vi "pcfs_signal_internal_stop.vi"(8 "error in (no error)":errorcluster, 11 "pcfs in":refnum<class "pcfs.lvclass">) -> (0 "error out":errorcluster, 3 "pcfs out":refnum<class "pcfs.lvclass">)   [LabVIEW 2015, in "pcfs.lvclass"]
uses:
  pcfs.lvclass
  pcfs_loop_notifier_tdef.ctl
  pcfs.lvclass/pcfs.ctl
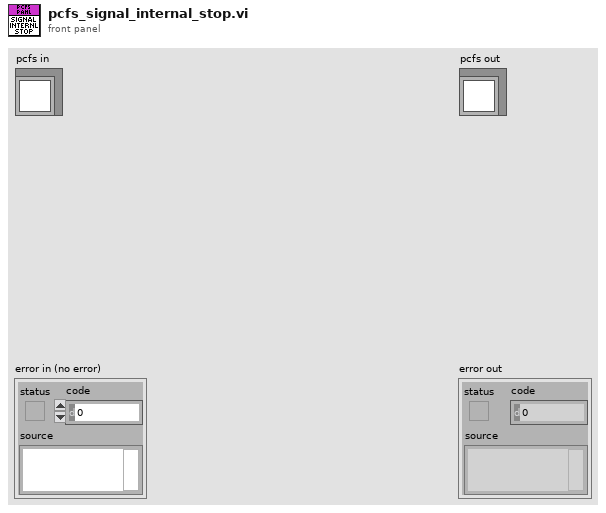
[diagram p1: front panel]
types:
  T1 = typedef "pcfs_loop_notifier_tdef.ctl" = enum16{"exit", "dither", "chart counts"}
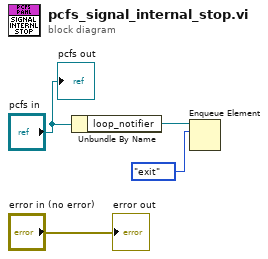
[diagram p0: block diagram]
diagram:
  n1 = Unbundle By Name("pcfs in") -> ("loop_notifier"=w2:refnum<queue>)
  n2 = Enqueue Element(queue=w2, element=pcfs_loop_notifier_tdef."exit") -> ()  [unwired: 2 in, 3 out]
  "error out" <- "error in (no error)"
  "pcfs out" <- "pcfs in"
